vi "Create Sequence.vi"(10 "Standard Config":string[][](array[string])=[["Simple", "", "", ""], ["Wait", "1000", "", ""], ["Update", "Boolean result 0", "Boolean", "True"], ["Wait ", "1000", "", ""], ["Update", "Boolean result 0", "Boolean", "False"]]) -> (2 "Sequence Config.lvclass":refnum<class "Sequence Config.lvclass">)   [LabVIEW 2015, in "Sequence Config.lvclass"]
uses:
  classes/Sequence Config/Sequence Config.lvclass
  classes/Wait Step Config/Wait Step Config.lvclass
  classes/Update Tag Step Config/Update Tag Configuration/Update Tag Config.lvclass
panel:
  out "error out":errorcluster
  in  "error in (no error)":errorcluster
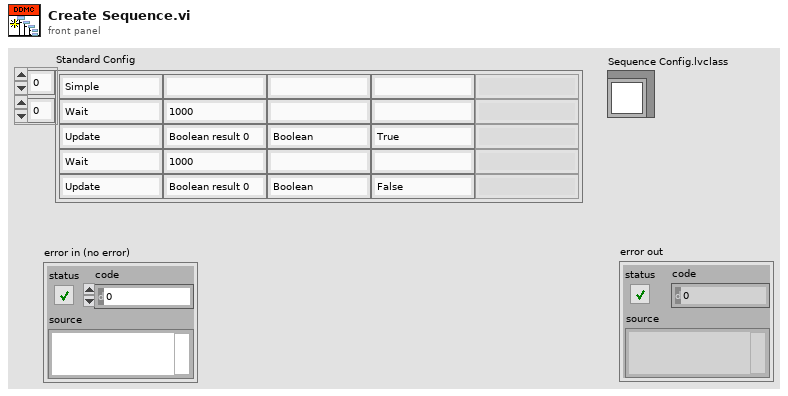
[diagram p1: front panel]
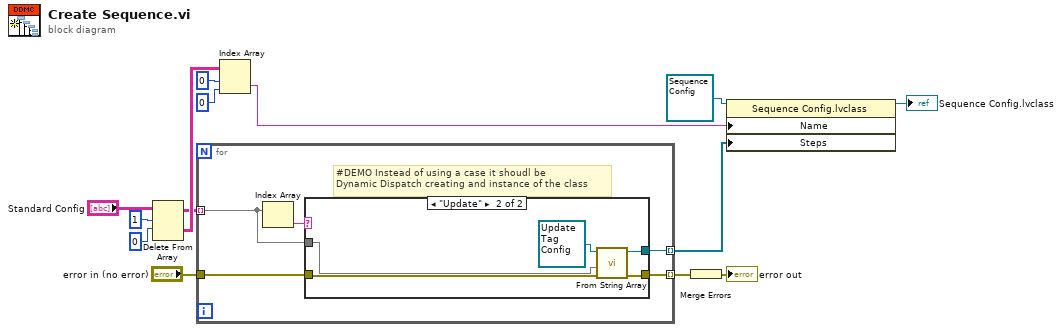
[diagram p0: block diagram]
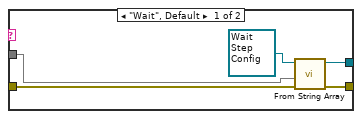
[diagram p2: hidden frame]
diagram:
  n1 = Delete From Array(array="Standard Config", length=1, index (row)=0) -> (deleted portion=w11:string[][], array with subset deleted=w9:string[][])  [unwired: 1 in]
  n2 = for {
    tunnel: w9 -> [w18] mode=indexing
    tunnel: "error in (no error)" -> [w16]
    tunnel: [w17] -> w3 mode=indexing
    tunnel: [w15] -> w2 mode=indexing
    # "#DEMO Instead of using a case it shoudl be\nDynamic Dispatch creating and instance of the class"
    n3 = Index Array(array=w18) -> (element=w19:string)  [unwired: 1 in]
    n4 = case shown="\"Update\"" w19 {
      tunnel: w18 -> [w22 w25]
      tunnel: [w23 w28] -> w17
      tunnel: w16 -> [w21 w26]
      tunnel: [w20 w27] -> w15
      frame "Wait", Default {
        n5 = call-dynamic "From String Array.vi"("error in (no error)"=w21, "String Array"=w22, "Wait Step Config in"=refnum<class "Wait Step Config.lvclass"> refnum ("Wait Step Config.lvclass")) -> ("error out"=w20:errorcluster, "Wait Step Config out"=w23:refnum<class "Wait Step Config.lvclass">)  [unwired: 7 in]
      }
      frame "Update" {
        n6 = call-dynamic "From String Array.vi"("error in (no error)"=w26, "String Array"=w25, "Update Tag Config in"=refnum<class "Update Tag Config.lvclass"> refnum ("Update Tag Config.lvclass")) -> ("error out"=w27:errorcluster, "Update Tag Config out"=w28:refnum<class "Update Tag Config.lvclass">)  [unwired: 7 in]
      }
    }
  }
  n7 = Index Array(array=w11, index (row)=0 ("index"), index (col)=0 ("disabled index (col)")) -> (element=w4:string)
  n8 = Merge Errors(w2) -> (→"error out":errorcluster)
  n9 = property class="Sequence Config.lvclass"(reference=refnum<class "Sequence Config.lvclass"> refnum ("Sequence Config.lvclass"), "Name"=w4, "Steps"=w3) -> (reference out=→"Sequence Config.lvclass":refnum<class "Sequence Config.lvclass">)  [unwired: 1 in, 1 out]
